vi "Get Max in Waveform Subset.vi"(11 "Pull-In Boost Waveform Section":dbl[](array[numeric])) -> (3 "Max":dbl)   [LabVIEW 2015, in "Fuel Injection Addon Engine.lvlib"]
uses:
  Fuel Injection Addon Engine.lvlib
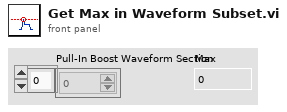
[diagram p1: front panel]
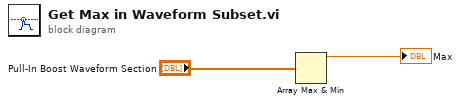
[diagram p0: block diagram]
diagram:
  n1 = Array Max & Min(array="Pull-In Boost Waveform Section") -> (max value=→"Max":dbl)  [unwired: 3 out]
